vi "svx_Polar_Draw_Circles.vi"(8 "grid measurements":T1 {"end angle" format="%.2f"; "start angle" format="%.2f"; "scale factors"."b" format="%.2f"; "scale factors"."a" format="%.2f"}, 9 "decade specs":cluster{"radius":i16, "label":string}[](array[cluster]), 11 "picture":picture) -> (3 "new picture":picture)   [LabVIEW 2017, in "SVX Polar Plot.xctl"]
uses:
  <vilib>/addons/_XControls/Polar Plot/SVX Polar Plot.xctl
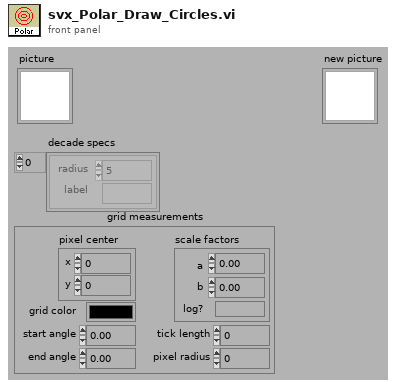
[diagram p1: front panel]
types:
  T1 = cluster{"pixel center":cluster{"x":i16, "y":i16}, "scale factors":cluster{"a":dbl, "b":dbl, "log?":bool}, "grid color":u32, "start angle":dbl, "end angle":dbl, "tick length":i16, "pixel radius":i32}
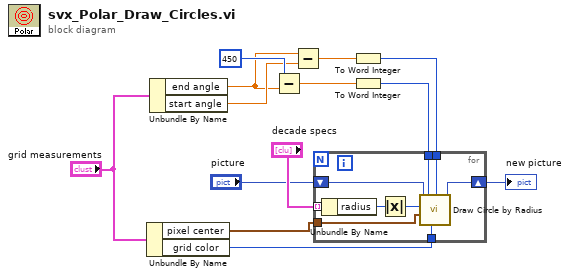
[diagram p0: block diagram]
diagram:
  n1 = Unbundle By Name("grid measurements") -> ("pixel center"=w11:cluster{"x":i16, "y":i16}, "grid color"=w12:u32)
  n2 = Unbundle By Name("grid measurements") -> ("end angle"=w5:dbl, "start angle"=w6:dbl)
  n3 = Subtract(x=450, y=w5) -> (x-y=w2:dbl)
  n4 = Subtract(x=w5, y=w6) -> (x-y=w4:dbl)
  n5 = To Word Integer(number=w4) -> (16bit integer=w3:i16)
  n6 = To Word Integer(number=w2) -> (16bit integer=w1:i16)
  n7 = for {
    tunnel: "decade specs" -> [w22] mode=indexing
    shift-right: [w19] -> w9
    shift-left: "picture" -> [w20]
    tunnel: w11 -> [w18]
    tunnel: w12 -> [w17]
    tunnel: w1 -> [w16]
    tunnel: w3 -> [w15]
    n8 = Unbundle By Name(w22) -> ("radius"=w21:i16)
    n9 = Absolute Value(x=w21) -> (abs(x)=w14:i16)
    n10 = call <vilib>:"Draw Circle by Radius.vi"("arc size(360)"=w15, "color(black)"=w17, "start angle(0)"=w16, "pixel center"=w18, "radius"=w14, "picture"=w20) -> ("new picture"=w19:picture)  [unwired: 5 in]
  }
  "new picture" <- w9
